vi "getImages.vi"(6 "Array":dbl[](array[numeric]), 7 "ROI 2":i32[][](array[numeric]), 9 "number of cam":i32=3, 10 "data":T1, 11 "SubscriberCluster":T5) -> (0 "B[mT]":dbl, 1 "Images":T7, 2 "ROI":T3, 3 "OK":bool[](array[boolean]), 4 "Numeric":u32, 5 "image ok":bool[](array[boolean]))   [LabVIEW 2013, in "MagAnalysis_Online.lvclass"]
uses:
  MagAnalysis_Online.lvclass
  ROIStartfromCam_typdef.ctl
  classicROI_typDef.ctl
  analysis_data_typdef.ctl
  <vilib>/vision/Image Controls.llb/IMAQ Image.ctl
  dataTypdef.ctl
  shared/SubscriberCluster_TypDEf.ctl
  Interface/Sandbox/GUI_Template/GUI_master/tcp_new_data_event.ctl
  Interface/Sandbox/GUI_Template/GUI_master/tcp new data cluster.ctl
  <vilib>/vision/NI_Vision_Development_Module.lvlib
panel:
  out "data 2":T1
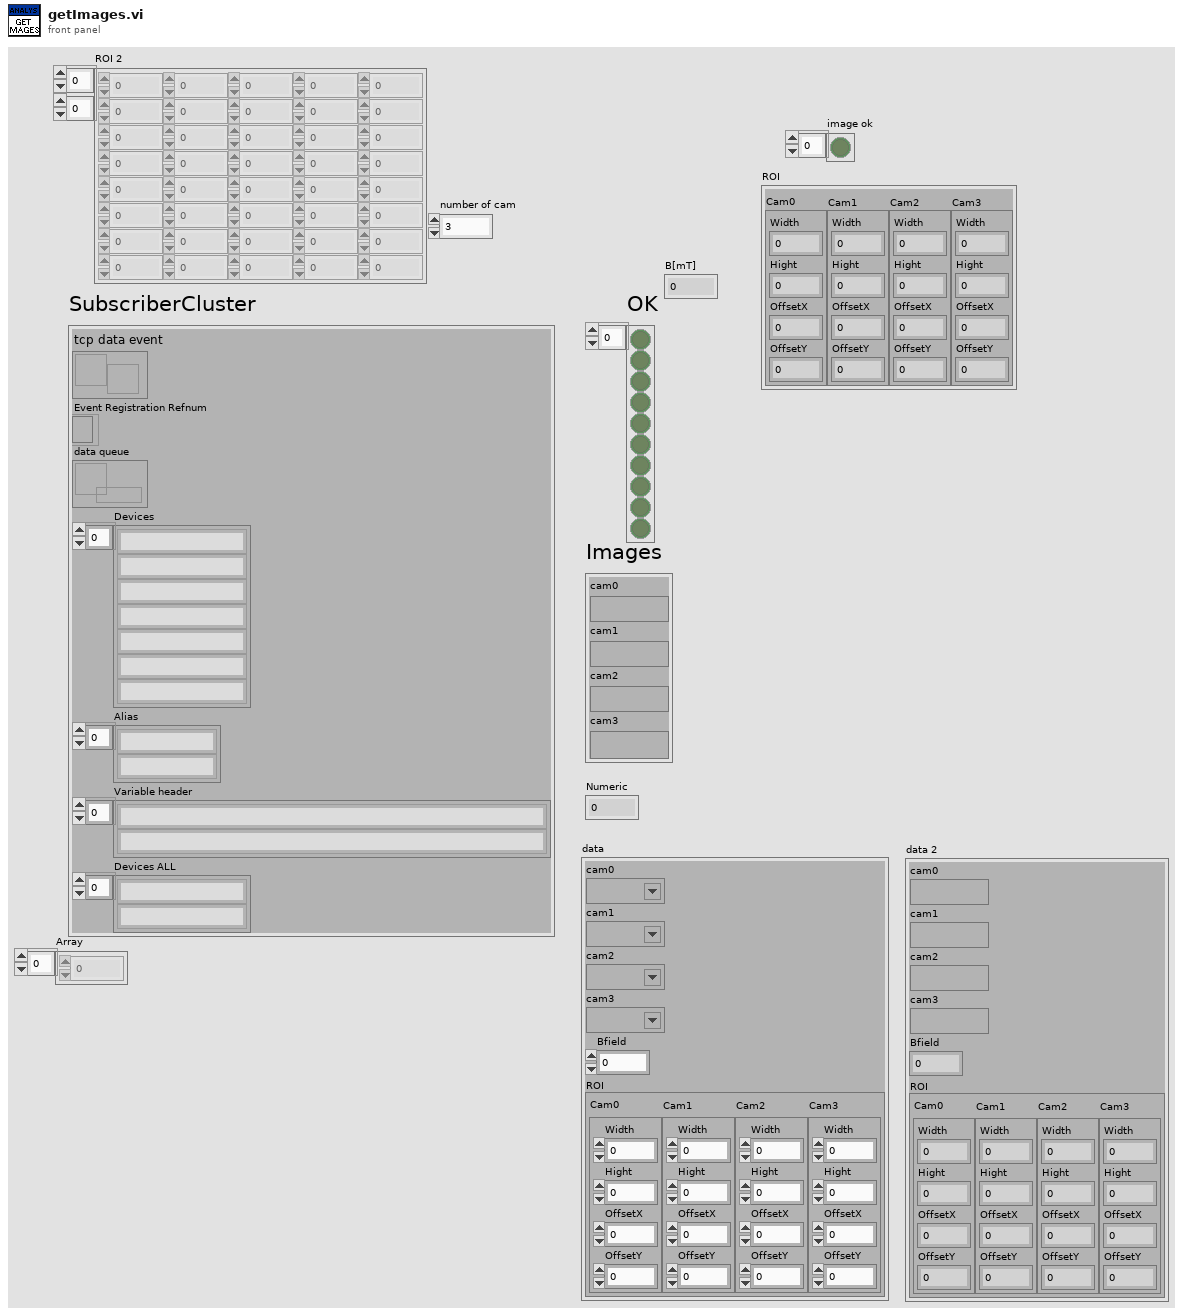
[diagram p1: front panel]
types:
  T1 = typedef "dataTypdef.ctl" = cluster{"cam0":T2, "cam1":T2, "cam2":T2, "cam3":T2, "Bfield":dbl, "ROI":T3}
  T2 = typedef "IMAQ Image.ctl" = refnum<image>
  T3 = typedef "ROIStartfromCam_typdef.ctl" = cluster{"Cam0":T4, "Cam1":T4, "Cam2":T4, "Cam3":T4}
  T4 = typedef "classicROI_typDef.ctl" = cluster{"Width":dbl, "Hight":dbl, "OffsetX":dbl, "OffsetY":dbl}
  T5 = typedef "SubscriberCluster_TypDEf.ctl" = cluster{"tcp data event":T6, "Event Registration Refnum":refnum<event-registration>, "data queue":refnum<queue>, "Devices":string[], "Alias":string[], "Variable header":string[], "Devices ALL":string[]}
  T6 = typedef "tcp_new_data_event.ctl" = refnum<user-event>
  T7 = typedef "MagAnalysis_Online.lvclass/analysis_data_typdef.ctl" = cluster{"cam0":T2, "cam1":T2, "cam2":T2, "cam3":T2}
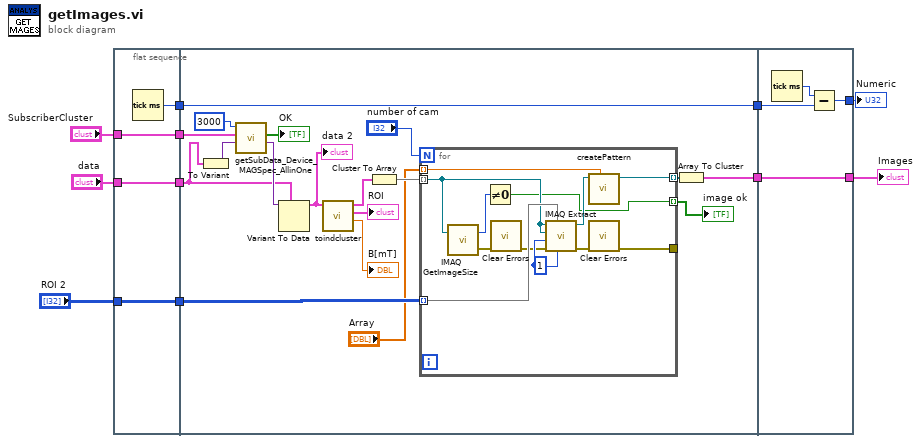
[diagram p0: block diagram]
diagram:
  n1 = flat-sequence {
    tunnel: "data" -> [w14]
    tunnel: "SubscriberCluster" -> [w15]
    tunnel: [w15] -> w11
    tunnel: [w14] -> w10
    tunnel: [w13] -> w9
    tunnel: "ROI 2" -> [w12]
    tunnel: [w12] -> w1
    tunnel: [w22] -> w8
    tunnel: w11 -> [w33]
    tunnel: w10 -> [w17]
    tunnel: w9 -> [w28]
    tunnel: [w28] -> w7
    tunnel: w1 -> [w19]
    tunnel: [w49] -> w4
    tunnel: w8 -> [w49]
    tunnel: w7 -> [w47]
    tunnel: [w46] -> w6
    frame #0 {
      n2 = Tick Count (ms)() -> (millisecond timer value=w13:u32)
    }
    frame #1 {
      n3 = To Variant(anything=w17) -> (Variant=w16:variant)
      n4 = call "getSubData_Device_MAGSpec_AllinOne.vi"("variant in"=w16, "SubscriberCluster"=w33, "timeout"=3000) -> ("variant out"=w31:variant, "OK"=→"OK":bool[])  [unwired: 7 in]
      n5 = Variant To Data(type=w17, Variant=w31) -> (data=w26:T1)  [unwired: 1 in, 1 out]
      "data 2" <- w26
      n6 = call "toindcluster.vi"("data"=w26) -> ("B[mT]"=→"B[mT]":dbl, "ROI"=→"ROI":T3, "Images"=w25:T7)  [unwired: 8 in]
      n7 = Cluster To Array(cluster=w25) -> (array=w24:T2[])
      n8 = for {
        N: "number of cam" -> [_]
        tunnel: w24 -> [w39] mode=indexing
        tunnel: w19 -> [w45] mode=indexing
        tunnel: [w42] -> w23 mode=indexing
        tunnel: [w44] -> _
        tunnel: [w35] -> w20 mode=indexing
        tunnel: "Array" -> [w34] mode=indexing
        w37 = 1 ("Y Step Size")
        n9 = call "IMAQ GetImageSize"("Image"=w39) -> ("Y Resolution"=w40:i32, "error out"=w41:errorcluster)  [unwired: 3 in, 1 out]
        n10 = Not Equal To 0?(x=w40) -> (x != 0?=w35:bool)
        n11 = call <vilib>:"Clear Errors.vi"("error in (no error)"=w41) -> ("error out"=w36:errorcluster)  [unwired: 6 in]
        n12 = call "IMAQ Extract"("Y Step Size"=w37, "Optional Rectangle"=w45, "error in (no error)"=w36, "X Step Size"=w37, "Image Dst"=w39, "Image Src"=w39) -> ("error out"=w38:errorcluster, "Image Dst Out"=w43:T2)  [unwired: 4 in]
        n13 = call "createPattern.vi"("Numeric"=w34, "Refnum in"=w43) -> ("Image Out 3"=w42:T2)  [unwired: 9 in]
        n14 = call <vilib>:"Clear Errors.vi"("error in (no error)"=w38) -> ("error out"=w44:errorcluster)  [unwired: 6 in]
      }
      "image ok" <- w20
      n15 = Array To Cluster(array=w23) -> (cluster=w22:cluster{"[0]":T2, "[1]":T2, "[2]":T2, "[3]":T2})
    }
    frame #2 {
      n16 = Tick Count (ms)() -> (millisecond timer value=w48:u32)
      n17 = Subtract(x=w48, y=w47) -> (x-y=w46:u32)
    }
  }
  "Numeric" <- w6
  "Images" <- w4
